vi "Is Error.vi"(11 "Base Event Actor in":refnum<class "Base Event Actor.lvclass">) -> (3 "Base Event Actor out":refnum<class "Base Event Actor.lvclass">)   [LabVIEW 2021, in "jettl.lvlib" / "Base Event Actor.lvclass"]
uses:
  Base Event Actor.lvclass
  Event State/Error Event State/Error Event State.lvclass
  C:/git/jettl/src/jettl/Event State/Event State/Event State.lvclass
  Base Event Actor.lvclass/Base Event Actor.ctl
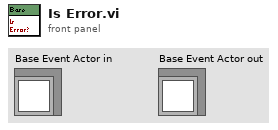
[diagram p1: front panel]
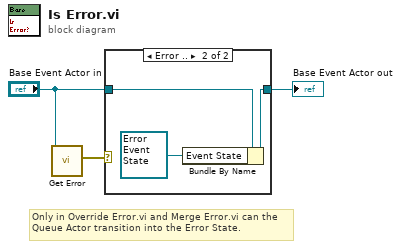
[diagram p0: block diagram]
diagram:
  # "Only in Override Error.vi and Merge Error.vi can the Queue Actor transition into the Error State."
  n1 = call-dynamic "Get Error.vi"("Base Event Actor in"="Base Event Actor in") -> ("Error"=w1:errorcluster)  [unwired: 10 in]
  n2 = case shown="Error .." w1 {
    tunnel: [w4 w6] -> w3
    tunnel: "Base Event Actor in" -> [w4 w7]
    frame No Error {
    }
    frame Error {
      n3 = Bundle By Name(cluster=w7, "Event State"=refnum<class "Error Event State.lvclass"> refnum ("jettl.lvlib:Error Event State.lvclass")) -> (w6:refnum<class "Base Event Actor.lvclass">)
    }
  }
  "Base Event Actor out" <- w3
